vi "IsLogTimerTriggered.vi"(11 "Timer (sec)":dbl) -> (3 "Triggered?":bool)   [LabVIEW 2013]
uses:
  LogStartTimeGlobalAction.ctl
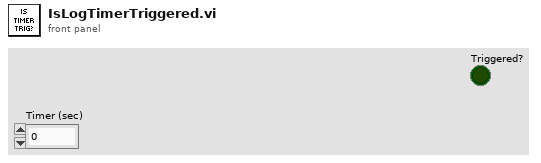
[diagram p1: front panel]
types:
  T1 = typedef "LogStartTimeGlobalAction.ctl" = enum16{"Set", "Get"}
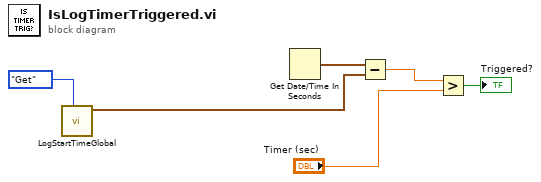
[diagram p0: block diagram]
diagram:
  n1 = call "LogStartTimeGlobal.vi"("Action"=LogStartTimeGlobalAction."Get") -> ("Value Out"=w1:timestamp)  [unwired: 10 in]
  n2 = Get Date/Time In Seconds() -> (seconds since 1Jan1904=w6:timestamp)
  n3 = Subtract(x=w6, y=w1) -> (x-y=w5:dbl)
  n4 = Greater?(x=w5, y="Timer (sec)") -> (0:→"Triggered?":bool)
